vi "Main.vi"(8 "error in (no error)":errorcluster, 11 "Plugin Thread in":refnum<class "Plugin Thread.lvclass">) -> (0 "error out":errorcluster, 3 "Plugin Thread out":refnum<class "Plugin Thread.lvclass">)   [LabVIEW 2017, in "DSF Core.lvlib" / "Plugin Thread.lvclass"]
uses:
  Thread/Plugin/Plugin Thread.lvclass
  Thread/Plugin/Plugin Thread.lvclass/Plugin Thread.ctl
  Interfaces/Interface/Interface.lvclass/Interface.ctl
  Transfer Group/Transfer Group.lvclass/Transfer Group.ctl
  Timing/Timing.lvclass/Timing.ctl
  Thread Pool/Pool.lvclass/Pool.ctl
  Interfaces/Plugin/Wait For.vi
  Interfaces/Plugin/Wait For Plugin Command.vi
  Get Interface.vi
  Cast Command to Transfer Group.vi
  Get Transfer Group by ID.vi
  Transfer Group/Set Current Iteration.vi
  Transfer Group/Write Return FIFO.vi
  Transfer Group/Get Thread.vi
  Thread Pool/Return Plugin Interface.vi
  Interfaces/Interface/Wait For Command.vi
  Get Transfer Group.vi
  Timing/Reset Iteration.vi
  Transfer Group/Get Timing.vi
  Timing/Get Iteration.vi
  Thread Pool/Write FIFO.vi
  Interfaces/Interface/Get ID.vi
  Interfaces/Interface/Read RT FIFO.vi
  Timing/Set Iteration.vi
  Interfaces/Plugin/Plugin Interface.lvclass
  C:/Git/DSF/Data Sharing Framework/Source/Core/Classes/Interfaces/Interface/Interface.lvclass
  Thread Pool/Plugin Interface Pool.lvclass
  C:/Git/DSF/Data Sharing Framework/Source/Core/Classes/Thread Pool/Pool.lvclass
  Interfaces/Plugin/Class Name.vi
  VIs/VI Name.vi
  Interfaces/Interface/Errors.vi
  Interfaces/Dispatcher/Command Timeout.vi
  Transceiver.lvclass
  Buffer Converter/Buffer Converter.lvclass
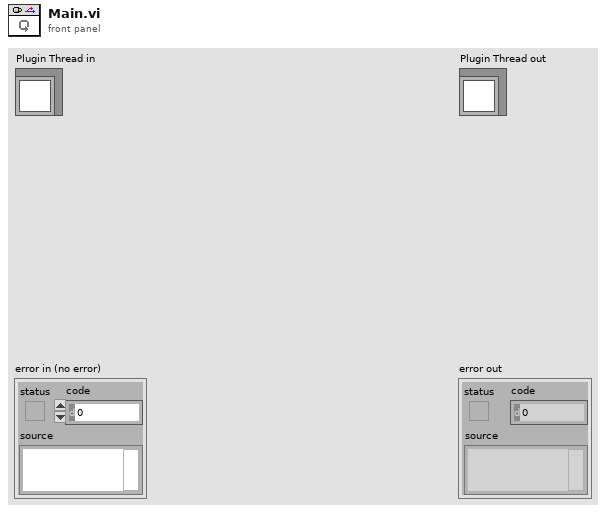
[diagram p1: front panel]
types:
  T1 = typedef "DSF Core.lvlib/Plugin Interface.lvclass/Command Data.ctl" = cluster{"Command":T2, "Parameters":T3}
  T2 = typedef "DSF Core.lvlib/Plugin Interface.lvclass/Command.ctl" = enum8{"Set Inline Buffer", "Rx", "Tx", "Shutdown"}
  T3 = typedef "DSF Core.lvlib/Plugin Interface.lvclass/Command Parameters.ctl" = cluster{"arg1":u64, "arg2":u64}
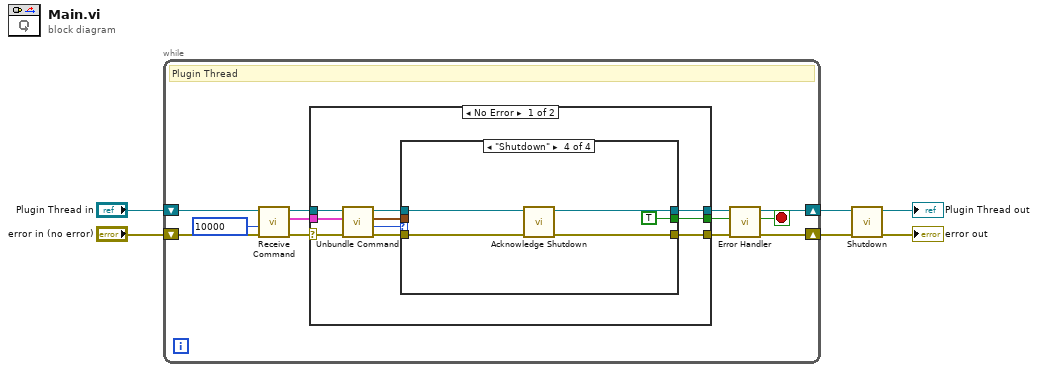
[diagram p0: block diagram]
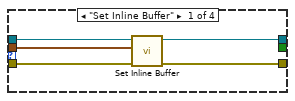
[diagram p2: hidden frame]
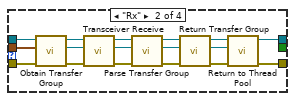
[diagram p3: hidden frame]
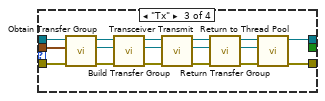
[diagram p4: hidden frame]
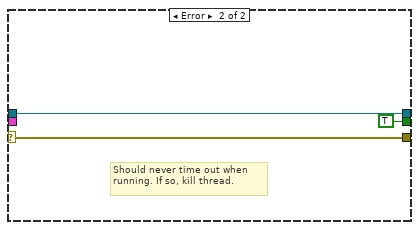
[diagram p5: hidden frame]
diagram:
  n1 = while {
    shift-right: [w13] -> w3
    shift-left: "error in (no error)" -> [w18]
    shift-right: [w14] -> w4
    shift-left: "Plugin Thread in" -> [w17]
    stop <- w12 stop-if-true
    # "Plugin Thread"
    n2 = call "Receive Command.vi"("error in (no error)"=w18, "timeout in ms (0)"=10000 ("timeout in ms"), "Plugin Thread in"=w17) -> ("error out"=w7:errorcluster, "command"=w8:T1, "Plugin Thread out"=w9:refnum<class "Plugin Thread.lvclass">)  [unwired: 6 in]
    n3 = case shown="No Error" w7 {
      selector: w7 -> [w19 w73]
      tunnel: w9 -> [w26 w75]
      tunnel: [w28 w75] -> w16
      tunnel: w8 -> [w25 _]
      tunnel: [w27 w73] -> w15
      tunnel: [w20 TRUE] -> w11
      frame No Error {
        n4 = call "Unbundle Command.vi"("error in (no error)"=w19, "command"=w25, "Plugin Thread in"=w26) -> ("error out"=w23:errorcluster, "command"=w24:T2, "command parameters"=w21:T3, "Plugin Thread out"=w22:refnum<class "Plugin Thread.lvclass">)  [unwired: 5 in]
        n5 = case shown="\"Shutdown\"" w24 {
          tunnel: w22 -> [w33 w40 w57 w72]
          tunnel: [w32 w42 w60 w70] -> w28
          tunnel: w23 -> [w29 w35 w56 w71]
          tunnel: w21 -> [w30 w39 w53 _]
          tunnel: [w31 w41 w59 w69] -> w27
          tunnel: [_ _ _ TRUE] -> w20
          frame "Set Inline Buffer" {
            n6 = call "Set Inline Buffer.vi"("error in (no error)"=w29, "command parameters"=w30, "Plugin Thread in"=w33) -> ("error out"=w31:errorcluster, "Plugin Thread out"=w32:refnum<class "Plugin Thread.lvclass">)  [unwired: 7 in]
          }
          frame "Rx" {
            n7 = call "Obtain Transfer Group.vi"("error in (no error)"=w35, "command parameters"=w39, "Transceiver Thread in"=w40) -> ("error out"=w37:errorcluster, "Transfer Group"=w36:refnum<class "Transfer Group.lvclass">, "Transceiver Thread out"=w38:refnum<class "Plugin Thread.lvclass">)  [unwired: 6 in]
            n8 = call "Transceiver Receive.vi"("error in (no error)"=w37, "Transfer Group in"=w36, "Transceiver Thread in"=w38) -> ("error out"=w49:errorcluster, "Transfer Group out"=w48:refnum<class "Transfer Group.lvclass">, "Transceiver Thread out"=w50:refnum<class "Plugin Thread.lvclass">)  [unwired: 6 in]
            n9 = call "Parse Transfer Group.vi"("error in (no error)"=w49, "Transfer Group in"=w48, "Plugin Thread in"=w50) -> ("error out"=w46:errorcluster, "Transfer Group out"=w45:refnum<class "Transfer Group.lvclass">, "Plugin Thread out"=w47:refnum<class "Plugin Thread.lvclass">)  [unwired: 6 in]
            n10 = call "Return Transfer Group.vi"("error in (no error)"=w46, "Transfer Group in"=w45, "Transceiver Thread in"=w47) -> ("error out"=w43:errorcluster, "Transfer Group out"=w34:refnum<class "Transfer Group.lvclass">, "Transceiver Thread out"=w44:refnum<class "Plugin Thread.lvclass">)  [unwired: 6 in]
            n11 = call "Return to Thread Pool.vi"("error in (no error)"=w43, "Transfer Group in"=w34, "Plugin Thread in"=w44) -> ("error out"=w41:errorcluster, "Plugin Thread out"=w42:refnum<class "Plugin Thread.lvclass">)  [unwired: 7 in]
          }
          frame "Tx" {
            n12 = call "Obtain Transfer Group.vi"("error in (no error)"=w56, "command parameters"=w53, "Transceiver Thread in"=w57) -> ("error out"=w54:errorcluster, "Transfer Group"=w52:refnum<class "Transfer Group.lvclass">, "Transceiver Thread out"=w55:refnum<class "Plugin Thread.lvclass">)  [unwired: 6 in]
            n13 = call "Build Transfer Group.vi"("error in (no error)"=w54, "Transfer Group in"=w52, "Plugin Thread in"=w55) -> ("error out"=w66:errorcluster, "Transfer Group out"=w58:refnum<class "Transfer Group.lvclass">, "Plugin Thread out"=w67:refnum<class "Plugin Thread.lvclass">)  [unwired: 6 in]
            n14 = call "Transceiver Transmit.vi"("error in (no error)"=w66, "Transfer Group in"=w58, "Transceiver Thread in"=w67) -> ("error out"=w64:errorcluster, "Transfer Group out"=w63:refnum<class "Transfer Group.lvclass">, "Transceiver Thread out"=w65:refnum<class "Plugin Thread.lvclass">)  [unwired: 6 in]
            n15 = call "Return Transfer Group.vi"("error in (no error)"=w64, "Transfer Group in"=w63, "Transceiver Thread in"=w65) -> ("error out"=w61:errorcluster, "Transfer Group out"=w51:refnum<class "Transfer Group.lvclass">, "Transceiver Thread out"=w62:refnum<class "Plugin Thread.lvclass">)  [unwired: 6 in]
            n16 = call "Return to Thread Pool.vi"("error in (no error)"=w61, "Transfer Group in"=w51, "Plugin Thread in"=w62) -> ("error out"=w59:errorcluster, "Plugin Thread out"=w60:refnum<class "Plugin Thread.lvclass">)  [unwired: 7 in]
          }
          frame "Shutdown" {
            n17 = call "Acknowledge Shutdown.vi"("error in (no error)"=w71, "Plugin Thread in"=w72) -> ("error out"=w69:errorcluster, "Plugin Thread out"=w70:refnum<class "Plugin Thread.lvclass">)  [unwired: 8 in]
          }
        }
      }
      frame Error {
        # "Should never time out when running. If so, kill thread."
      }
    }
    n18 = call "Error Handler.vi"("error in (no error)"=w15, "stop"=w11, "Plugin Thread in"=w16) -> ("error out"=w13:errorcluster, "stop"=w12:bool, "Plugin Thread out"=w14:refnum<class "Plugin Thread.lvclass">)  [unwired: 6 in]
  }
  n19 = call "Shutdown"("error in (no error)"=w3, "Plugin Thread in"=w4) -> ("error out"=→"error out":errorcluster, "Plugin Thread out"=→"Plugin Thread out":refnum<class "Plugin Thread.lvclass">)  [unwired: 8 in]
